vi "unsubscribeParam.vi"(8 "error in":errorcluster, 11 "Node ROS":T1={"topic port"=0, "Node"="", "topic"="", "type"="", "node port"=0, "error "={"status"=FALSE, "code"=0, "source"=""}, "Direction"=enum."Node", "APIs"=[], "Update (ms)"=1, "write queue"=1}) -> (0 "error out":errorcluster, 2 "XML Received":string, 3 "Node ROS Out":T1={"topic port"=0, "Node"="", "topic"="", "type"="", "node port"=0, "error "={"status"=FALSE, "code"=0, "source"=""}, "Direction"=enum."Node", "APIs"=[], "Update (ms)"=1, "write queue"=1})   [LabVIEW 2012]
doc: "Reads a parameter from the parameter server. The parameter server must be running at the same address as the ROS master."
uses:
  <userlib>/ROSforLV/ROS/Code/SubVIs/_ROSControl.ctl
  <userlib>/ROSforLV/ROS/Code/SubVIs/_ROSDirection.ctl
panel:
  out "resulting string":string
  in  "parameter name":string
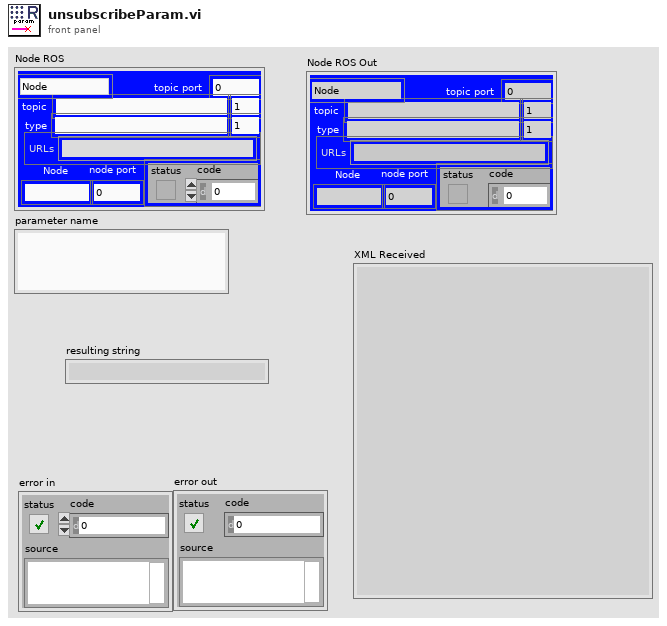
[diagram p1: front panel]
types:
  T1 = typedef "_ROSControl.ctl" = cluster{"topic port":u16, "Node":string, "topic":string, "type":string, "node port":u32, "error ":errorcluster, "Direction":T2, "APIs":string[], "Update (ms)":u16, "write queue":u16}
  T2 = typedef "_ROSDirection.ctl" = enum16{"Node", "Publisher", "Subscriber", "Service Client"}
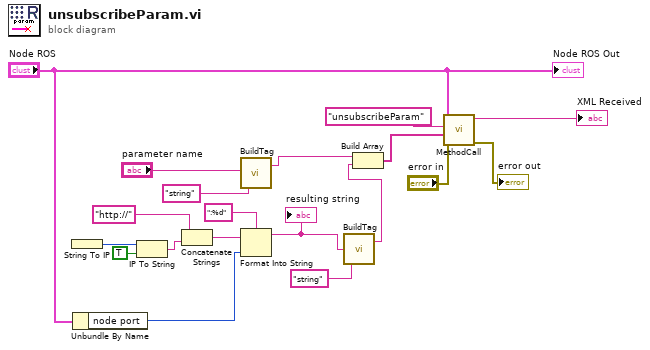
[diagram p0: block diagram]
diagram:
  n1 = String To IP() -> (0:w8:u32)  [unwired: 1 in]
  n2 = Unbundle By Name("Node ROS") -> ("node port"=w1:u32)
  n3 = IP To String(1:TRUE ("dot notation? (F)"), 2:w8) -> (0:w4:string)
  n4 = Concatenate Strings("http://" ("string"), w4) -> (w2:string)
  n5 = call <userlib>:"BuildTag.vi"("tag"="string", "value"="parameter name") -> ("string out"=w13:string)  [unwired: 2 in]
  n6 = Format Into String(format string=":%d", initial string=w2, w1) -> (resulting string=w5:string)  [unwired: 1 in, 1 out]
  "resulting string" <- w5
  n7 = call <userlib>:"BuildTag.vi"("tag"="string", "value"=w5) -> ("string out"=w11:string)  [unwired: 2 in]
  n8 = Build Array(w13, w11) -> (w12:string[])
  n9 = call <userlib>:"MethodCall.vi"("error in"="error in", "Method Params"=w12, "methodName"="unsubscribeParam", "Node ROS"="Node ROS") -> ("error out"=→"error out":errorcluster, "XML Received"=→"XML Received":string)  [unwired: 6 in]
  "Node ROS Out" <- "Node ROS"
